vi "Parce Request.vi"(8 "error in":errorcluster) -> (0 "error out":errorcluster, 3 "MES Request":string)   [LabVIEW 2023, in "MES.lvlib"]
uses:
  MES.lvlib
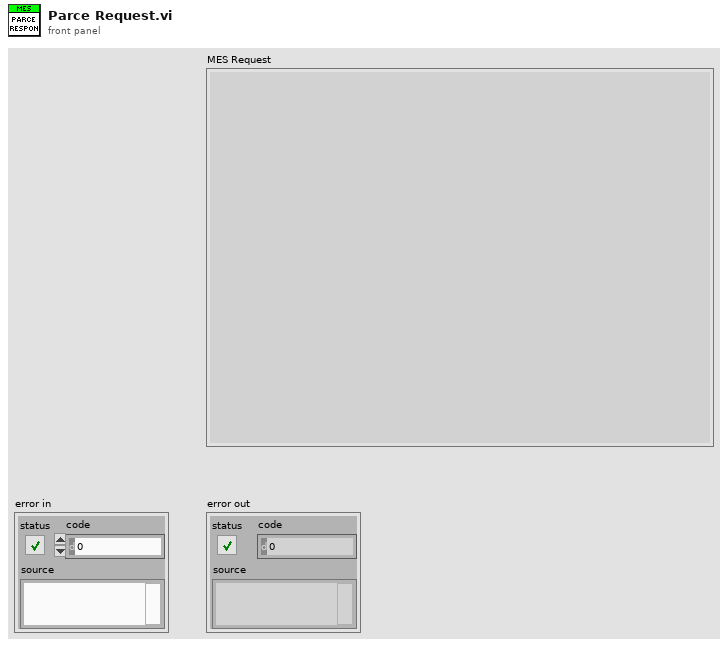
[diagram p1: front panel]
types:
  T1 = enum16{"open", "replace", "create", "open or create", "replace or create", "replace or create with confirmation"}
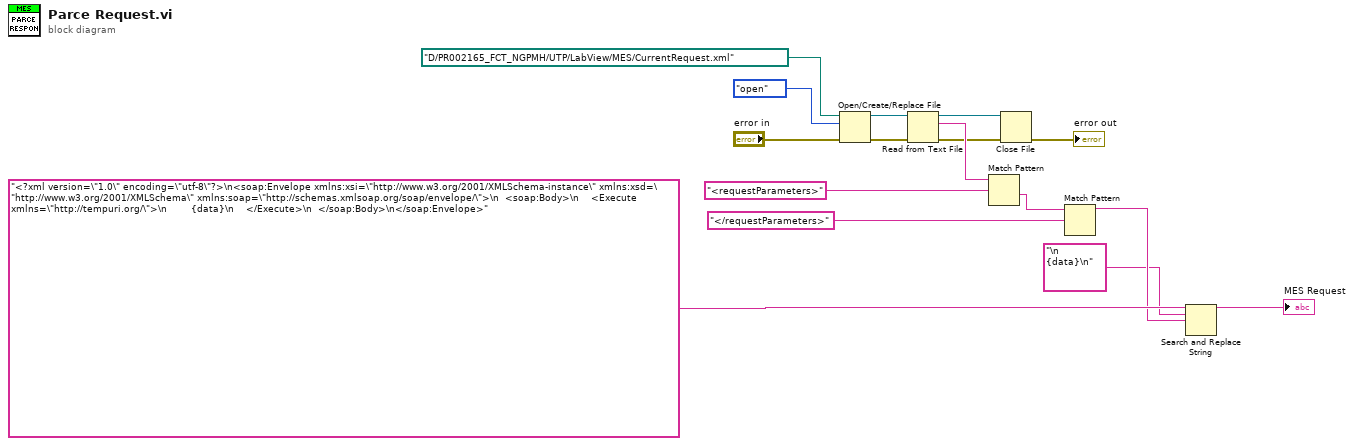
[diagram p0: block diagram]
diagram:
  n1 = Open/Create/Replace File(file path (use dialog)=path "D:/PR002165_FCT_NGPMH/UTP/LabView/MES/CurrentRequest.xml", error in="error in", operation (0:open)=T1."open") -> (refnum out=w16:refnum<file>, error out=w8:errorcluster)  [unwired: 3 in, 1 out]
  n2 = Read from Text File(file (use dialog)=w16, error in=w8) -> (refnum out=w12:refnum<file>, text=w15:string, error out=w7:errorcluster)  [unwired: 2 in, 1 out]
  n3 = Match Pattern(string=w15, regular expression="<requestParameters>") -> (after substring=w14:string)  [unwired: 1 in, 3 out]
  n4 = Close File(refnum=w12, error in=w7) -> (error out=→"error out":errorcluster)  [unwired: 1 out]
  n5 = Match Pattern(string=w14, regular expression="</requestParameters>") -> (before substring=w4:string)  [unwired: 1 in, 3 out]
  n6 = Search and Replace String(input string="<?xml version=\"1.0\" encoding=\"utf-8\"?>\n<soap:Envelope xmlns:xsi=\"http://www.w3.org/2001/XMLSchema-instance\" xmlns:xsd=\"http://www.w3.org/2001/XMLSchema\" xmlns:soap=\"http://schemas.xmlsoap.org/soap/envelope/\">\n  <soap:Body>\n    <Execute xmlns=\"http://tempuri.org/\">\n        {data}\n    </Execute>\n  </soap:Body>\n</soap:Envelope>" ("MES Response"), search string="\n        {data}\n", replace string=w4) -> (result string=→"MES Request":string)  [unwired: 5 in, 3 out]
